vi "Hallbar.vi"(8 "polynomial order":i32=2, 10 "R vs B":cluster{dbl[], dbl[]}[](graph)=[{array[8238 elements], array[8238 elements]}], 11 "Is this Rxy?":bool=TRUE) -> (1 "Polynomial fit":cluster{dbl[], dbl[]}[](graph), 2 "Linear fit":cluster{dbl[], dbl[]}[](graph), 3 "Data - fit":cluster{dbl[], dbl[]}[](graph), 4 "Polynomial residue":dbl, 6 "Linear fit slope":dbl[](array[numeric])=[-8.323259165456882])   [LabVIEW 2020]
uses:
  <userlib>/LevyLab/XY Utilities/subVIs/Linear Fit (multiple).vi
  <userlib>/LevyLab/XY Utilities/subVIs/Get X and Y (single).vi
  <userlib>/LevyLab/XY Utilities/subVIs/Zero Phase Lowpass Filter (multiple).vi
  <userlib>/LevyLab/XY Utilities/subVIs/Linear Fit (single).vi
  <userlib>/LevyLab/XY Utilities/subVIs/Zero Phase Lowpass Filter (single).vi
  <userlib>/LevyLab/XY Utilities/Swap X and Y.vi
  <userlib>/LevyLab/XY Utilities/subVIs/Swap X and Y (single).vi
  <vilib>/Analysis/6fits.llb/Linear Fit Intervals.vi
  <vilib>/Analysis/6fits.llb/Confidence Interval (Linear).vi
  <userlib>/LevyLab/XY Utilities/Private/Get X Array dx.vi
  <vilib>/Utility/error.llb/Error Cluster From Error Code.vi
  <vilib>/Analysis/3filter.llb/FIR Windowed Coefficients.vi
  <vilib>/Analysis/3filter.llb/Zero Phase Filter.vi
  <vilib>/Analysis/3filter.llb/Zero Phase Filter (DBL).vi
  <userlib>/LevyLab/XY Utilities/xy_utilities.lvlib
  <vilib>/Analysis/NI_AALPro.lvlib
panel:
  in  "cutoff period (data)":dbl=3e-05 format="%#_13g"
  out "Data - fit 2":cluster{dbl[], dbl[]}[](graph)
  out "intercepts":dbl[](array[numeric])=[-1.7804090620037338]
  # "Put false for Rxx"
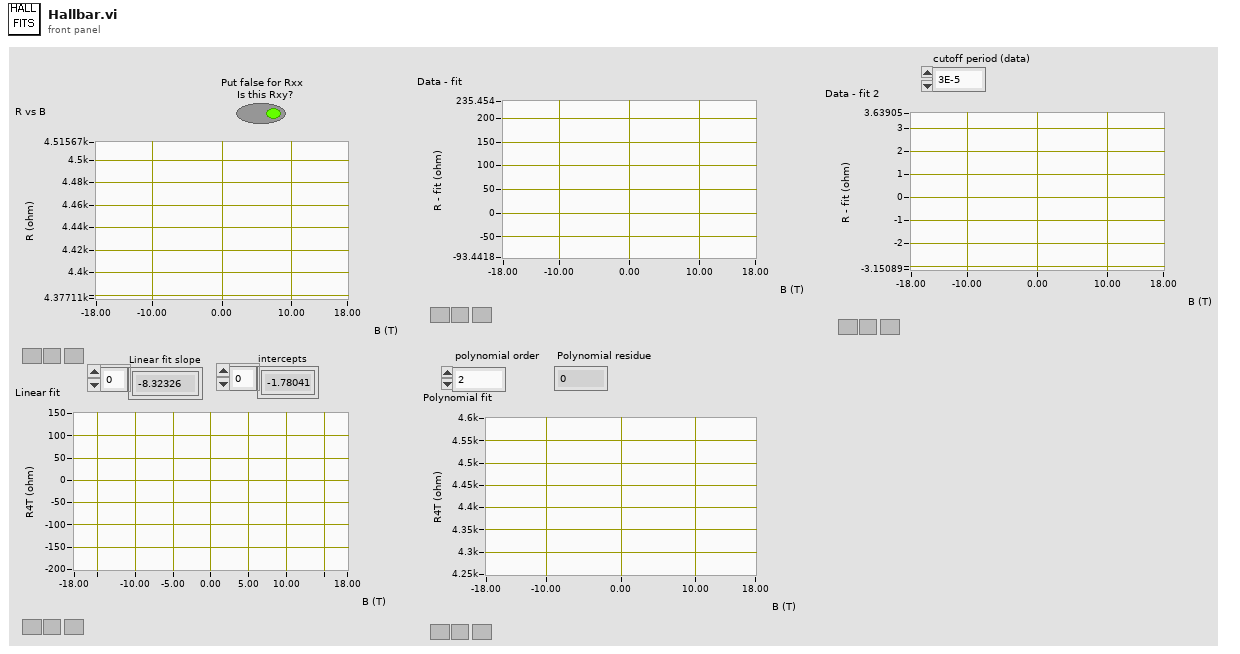
[diagram p1: front panel]
types:
  T1 = cluster{"X-array":dbl[], "Best Polynomial Fit":dbl[]}
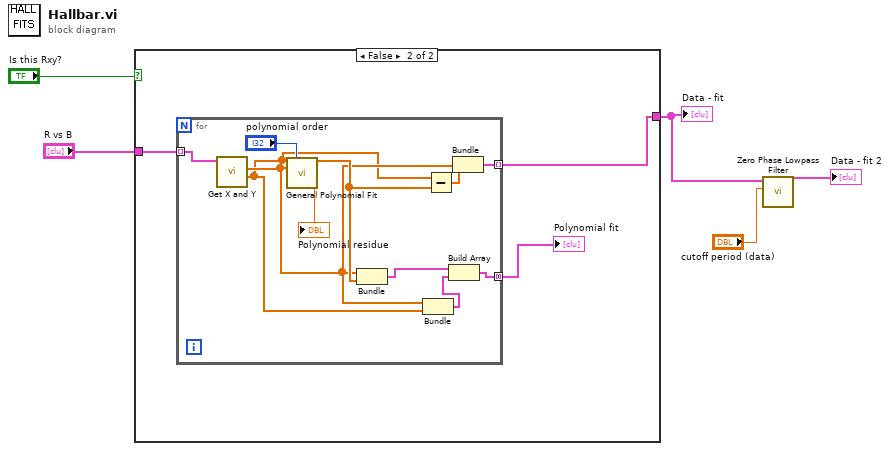
[diagram p0: block diagram]
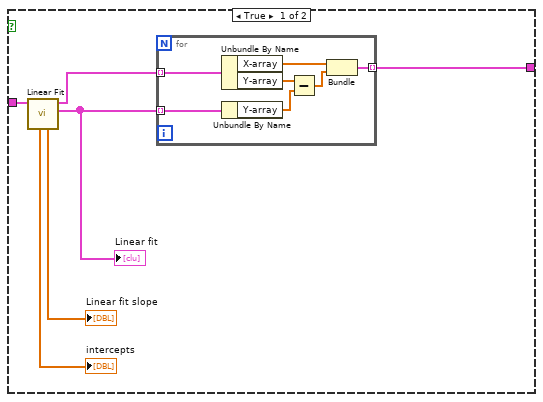
[diagram p2: hidden frame]
diagram:
  n1 = case shown="False" "Is this Rxy?" {
    tunnel: "R vs B" -> [w7 w21]
    tunnel: [w6 w19] -> w3
    frame True {
      n2 = call-poly <vilib>:"Linear Fit.vi"("XY-data"=w7) -> ("Best Fits"=w9:cluster{"X-array":dbl[], "Y-array":dbl[]}[], "XY-data out"=w8:cluster{"X-array":dbl[], "Y-array":dbl[]}[], "slopes"=→"Linear fit slope":dbl[], "intercepts"=→"intercepts":dbl[])  [unwired: 4 in, 3 out]
      "Linear fit" <- w9
      n3 = for {
        tunnel: w9 -> [w18] mode=indexing
        tunnel: w8 -> [w17] mode=indexing
        tunnel: [w13] -> w6 mode=indexing
        n4 = Unbundle By Name(w17) -> ("X-array"=w15:dbl[], "Y-array"=w12:dbl[])
        n5 = Unbundle By Name(w18) -> ("Y-array"=w16:dbl[])
        n6 = Subtract(x=w12, y=w16) -> (x-y=w14:dbl[])
        n7 = Bundle("X-array"=w15, w14) -> (w13:cluster{"X-array":dbl[], dbl[]})  [unwired: 1 in]
      }
    }
    frame False {
      n8 = for {
        tunnel: w21 -> [w32] mode=indexing
        tunnel: [w24] -> w20 mode=concatenating
        tunnel: [w28] -> w19 mode=indexing
        n9 = call-poly <userlib>:"Get X and Y.vi"("XY-data"=w32) -> ("Y-array"=w25:dbl[], "X-array"=w26:dbl[])  [unwired: 7 in, 2 out]
        n10 = call <vilib>:"General Polynomial Fit.vi"("Y"=w25, "polynomial order"="polynomial order", "X"=w26) -> ("Best Polynomial Fit"=w29:dbl[], "residue"=→"Polynomial residue":dbl)  [unwired: 9 in, 2 out]
        n11 = Bundle("X-array"=w26, "Best Polynomial Fit"=w29) -> (w22:T1)  [unwired: 1 in]
        n12 = Bundle("X-array"=w26, "Y-array"=w25) -> (w23:cluster{"X-array":dbl[], "Y-array":dbl[]})  [unwired: 1 in]
        n13 = Subtract(x=w25, y=w29) -> (x-y=w30:dbl[])
        n14 = Build Array(w22, w23) -> (w24:cluster{"X-array":dbl[], "Y-array":dbl[]}[])
        n15 = Bundle("X-array"=w26, w30) -> (w28:cluster{"X-array":dbl[], dbl[]})  [unwired: 1 in]
      }
      "Polynomial fit" <- w20
    }
  }
  "Data - fit" <- w3
  n16 = call-poly <userlib>:"Zero Phase Lowpass Filter.vi"("cutoff period (data)"="cutoff period (data)", "XY-data"=w3) -> ("XY-data out"=→"Data - fit 2":cluster{"X-array":dbl[], "Y-array":dbl[]}[])  [unwired: 8 in, 1 out]
